vi "Open Files.vi"(8 "error in (no error)":errorcluster, 11 "TimeStamper in":refnum<class "TimeStamper.lvclass">) -> (0 "error out":errorcluster, 3 "TimeStamper out":refnum<class "TimeStamper.lvclass">)   [LabVIEW 2014, in "TimeStamper.lvclass"]
uses:
  TimeStamper.lvclass
  TimeStamper.lvclass/TimeStamper.ctl
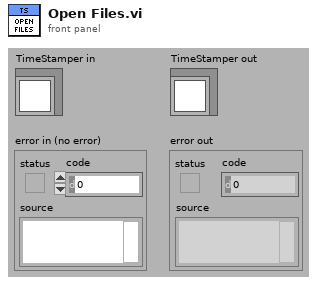
[diagram p1: front panel]
types:
  T1 = enum16{"open", "replace", "create", "open or create", "replace or create", "replace or create with confirmation"}
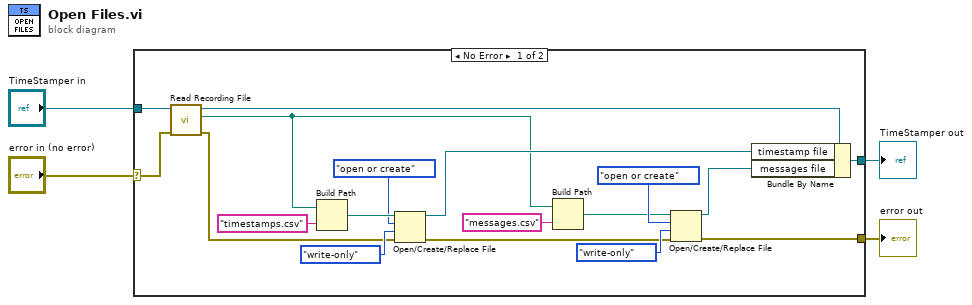
[diagram p0: block diagram]
diagram:
  n1 = case shown="No Error" "error in (no error)" {
    selector: "error in (no error)" -> [w12 w24]
    tunnel: [w10 w24] -> w3
    tunnel: [w6 w23] -> w1
    tunnel: "TimeStamper in" -> [w13 w23]
    frame No Error {
      n2 = call-dynamic "Read Recording File.vi"("error in (no error)"=w12, "AcquistionObject in"=w13) -> ("error out"=w11:errorcluster, "Recording File"=w5:path, "AcquistionObject out"=w7:refnum<class "TimeStamper.lvclass">)  [unwired: 7 in]
      n3 = Build Path(base path=w5, name or relative path="timestamps.csv") -> (appended path=w21:path)
      n4 = Open/Create/Replace File(file path (use dialog)=w21, error in=w11, operation (0:open)=T1."open or create", access (0:read/write)=enum16{"read/write", "read-only", "write-only"}."write-only") -> (refnum out=w9:refnum<file>, error out=w16:errorcluster)  [unwired: 2 in, 1 out]
      n5 = Build Path(base path=w5, name or relative path="messages.csv") -> (appended path=w14:path)
      n6 = Open/Create/Replace File(file path (use dialog)=w14, error in=w16, operation (0:open)=T1."open or create", access (0:read/write)=enum16{"read/write", "read-only", "write-only"}."write-only") -> (refnum out=w8:refnum<file>, error out=w10:errorcluster)  [unwired: 2 in, 1 out]
      n7 = Bundle By Name(cluster=w7, "timestamp file"=w9, "messages file"=w8) -> (w6:refnum<class "TimeStamper.lvclass">)
    }
    frame Error {
    }
  }
  "error out" <- w3
  "TimeStamper out" <- w1
